vi "Wait.vi"(7 "milliseconds to wait":u32, 11 "error in (no error)":errorcluster) -> (3 "error out":errorcluster)   [LabVIEW 2016, in "DronaTest.lvlib"]
uses:
  DronaTest.lvlib
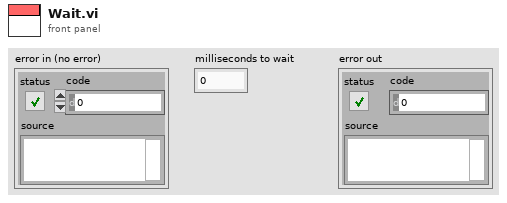
[diagram p1: front panel]
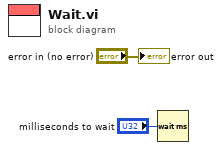
[diagram p0: block diagram]
diagram:
  n1 = Wait (ms)(milliseconds to wait="milliseconds to wait") -> ()  [unwired: 1 out]
  "error out" <- "error in (no error)"
